vi "EnableMotor.vi"(8 "error in (no error)":errorcluster, 10 "Axis (1) in":i32, 11 "VISA Refnum in":refnum<visa-resource-name>) -> (0 "error out":errorcluster, 3 "VISA Refnum out":refnum<visa-resource-name>)   [LabVIEW 2011]
uses:
  <instrlib>/Newport ESP301/Newport ESP301.lvlib
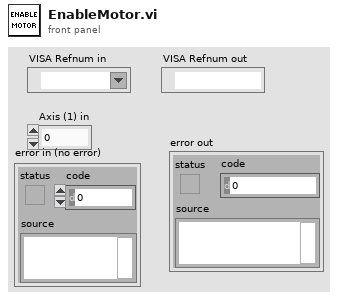
[diagram p1: front panel]
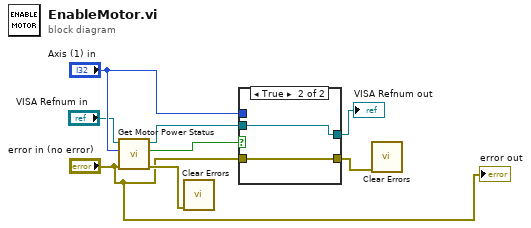
[diagram p0: block diagram]
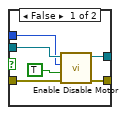
[diagram p2: hidden frame]
diagram:
  n1 = call <instrlib>:"Get Motor Power Status.vi"("error in (no error)"="error in (no error)", "Axis (1)"="Axis (1) in", "VISA resource name"="VISA Refnum in") -> ("error out"=w3:errorcluster, "Power Status"=w5:bool, "VISA resource name out"=w6:refnum<visa-resource-name>)  [unwired: 2 in]
  n2 = call <vilib>:"Clear Errors.vi"("error in (no error)"=w3) -> ()  [unwired: 6 in, 1 out]
  n3 = case shown="True" w5 {
    tunnel: w6 -> [w14 w16]
    tunnel: "Axis (1) in" -> [w13 _]
    tunnel: [w11 w16] -> w8
    tunnel: "error in (no error)" -> [w10 w15]
    tunnel: [w9 w15] -> w2
    frame False {
      n4 = call <instrlib>:"Enable Disable Motor.vi"("error in (no error)"=w10, "Action (OFF)"=TRUE, "Axis (1)"=w13, "VISA resource name"=w14) -> ("error out"=w9:errorcluster, "VISA resource name out"=w11:refnum<visa-resource-name>)  [unwired: 2 in]
    }
    frame True {
    }
  }
  "VISA Refnum out" <- w8
  n5 = call <vilib>:"Clear Errors.vi"("error in (no error)"=w2) -> ()  [unwired: 6 in, 1 out]
  "error out" <- "error in (no error)"
